vi "TestProcess.vi"(0 "VI Reference In":refnum<vi>, 5 "Wash Option":string, 7 "Car Position":u8=1, 9 "Elapsed Time":dbl=5.0, 11 "error in":errorcluster, 13 "Same Position?":bool) -> (4 "VI Reference Out":refnum<vi>, 15 "error out":errorcluster)   [LabVIEW 2016, in "CarWashTest.lvlib"]
uses:
  CarWashTest.lvlib
  APIs/Assert/AssertControlValue/False.vi
  APIs/Assert/AssertControlValue/True.vi
  APIs/Stimulus/ControlValue/SetValueAuto.vi
  APIs/Assert/AssertControlValue/Equal.vi
  APIs/Assert/AssertControlValue/AlmostEqual.vi
  <vilib>/addons/_JKI Toolkits/Caraya/classes/Test/Test.lvclass
  Drona.lvlib
  APIs/Assert/AssertControlValue/AssertControlValue.lvlib
  APIs/Stimulus/ControlValue/ControlValue.lvlib
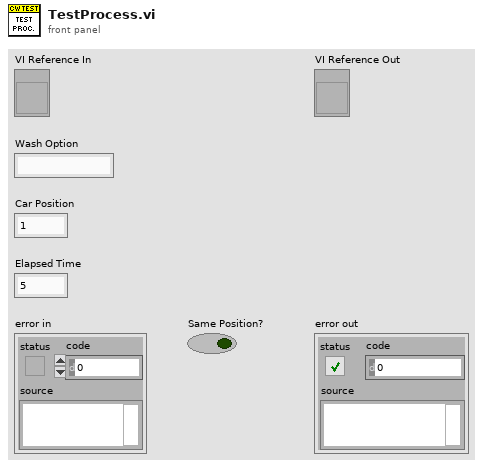
[diagram p1: front panel]
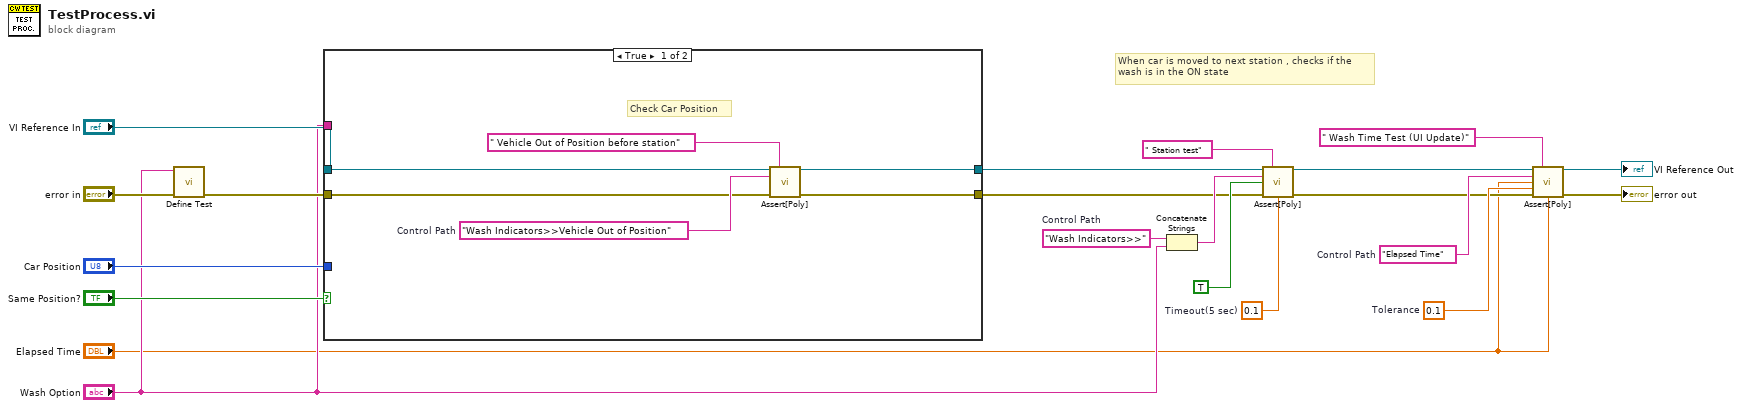
[diagram p0: block diagram]
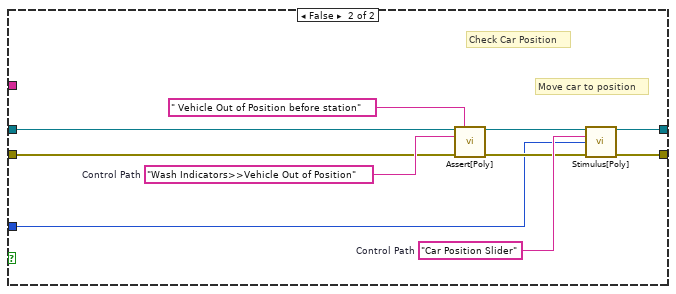
[diagram p2: hidden frame]
diagram:
  w12 = "Wash Indicators>>"  # Control Path
  w17 = 0.1  # Timeout(5 sec)
  w15 = 0.1  # Tolerance
  w16 = "Elapsed Time"  # Control Path
  # "When car is moved to next station , checks if the\nwash is in the ON state"
  n1 = call <vilib>:"Define Test.vi"("error in (no error)"="error in", "Label (VI Title)"="Wash Option") -> ("error out"=w8:errorcluster)  [unwired: 9 in]
  n2 = case shown="True" "Same Position?" {
    tunnel: [w24 w37] -> w9
    tunnel: [w23 w36] -> w13
    tunnel: "VI Reference In" -> [w26 w33]
    tunnel: w8 -> [w25 w31]
    tunnel: "Car Position" -> [_ w29]
    tunnel: "Wash Option" -> [_ _]
    frame True {
      w27 = "Wash Indicators>>Vehicle Out of Position"  # Control Path
      # "Check Car Position"
      n3 = call-poly "Assert[Poly].vi"("VI Reference In"=w26, "Label"=" Vehicle Out of Position before station", "Control Path"=w27, "Error In"=w25) -> ("VI Reference Out"=w23:refnum<vi>, "Error Out"=w24:errorcluster)  [unwired: 10 in]
    }
    frame False {
      w34 = "Wash Indicators>>Vehicle Out of Position"  # Control Path
      w35 = "Car Position Slider"  # Control Path
      # "Move car to position"
      # "Check Car Position"
      n4 = call-poly "Assert[Poly].vi"("VI Reference In"=w33, "Label"=" Vehicle Out of Position before station", "Control Path"=w34, "Error In"=w31) -> ("VI Reference Out"=w32:refnum<vi>, "Error Out"=w30:errorcluster)  [unwired: 10 in]
      n5 = call-poly "Stimulus[Poly].vi"("VI Reference In"=w32, "Control Path"=w35, "Value (Signaling)"=w29, "error in"=w30) -> ("VI Reference Out"=w36:refnum<vi>, "error out"=w37:errorcluster)  [unwired: 10 in]
    }
  }
  n6 = Concatenate Strings(w12, "Wash Option") -> (w11:string)
  n7 = call-poly "Assert[Poly].vi"("VI Reference In"=w13, "Label"=" Station test", "Control Path"=w11, "Control Value"=TRUE, "Error In"=w9, "Timeout(5 sec)"=w17) -> ("VI Reference Out"=w14:refnum<vi>, "Error Out"=w10:errorcluster)  [unwired: 8 in]
  n8 = call-poly "Assert[Poly].vi"("VI Reference In"=w14, "Label"=" Wash Time Test (UI Update)", "Control Path"=w16, "Control Value"="Elapsed Time", "Tolerance"=w15, "Error In"=w10, "Timeout(5 sec)"="Elapsed Time") -> ("VI Reference Out"=→"VI Reference Out":refnum<vi>, "Error Out"=→"error out":errorcluster)  [unwired: 7 in]
